vi "Pre Launch Init.vi"(11 "Keypad in":refnum<class "Keypad.lvclass">) -> (0 "error out":errorcluster, 3 "Keypad out":refnum<class "Keypad.lvclass">)   [LabVIEW 2020, in "Keypad.lvlib" / "Keypad.lvclass"]
doc: "(<B>Filename</B>: Actor Framework.lvlib:Actor.lvclass:Pre Launch Init.vi)\n\nDefines behavior that occurs after the Launch Actor method is invoked but before the actor's Actor Core method begins running.\n\nThe Pre Launch Init method is guaranteed to finish before the Launch Actor method returns to its caller and before the actor itself receives any messages. Any references that the Pre Launch Init method obtains are guaranteed to have the same lifetime as the actor itself. Any errors that the Pre Launch Init method returns will abort the launch.\n\nBy default, this method does nothing. A descendant class may override it to define behavior."
uses:
  Keypad.lvclass
  <vilib>/ni/Actors/State Actor/State Actor/State Actor.lvclass
  Type Def - Cursor Display.ctl
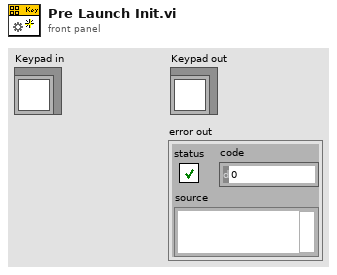
[diagram p1: front panel]
types:
  T1 = typedef "Type Def - Cursor Display.ctl" = cluster{"Up":bool, "Left":bool, "Ctr":bool, "Right":bool, "Down":bool}
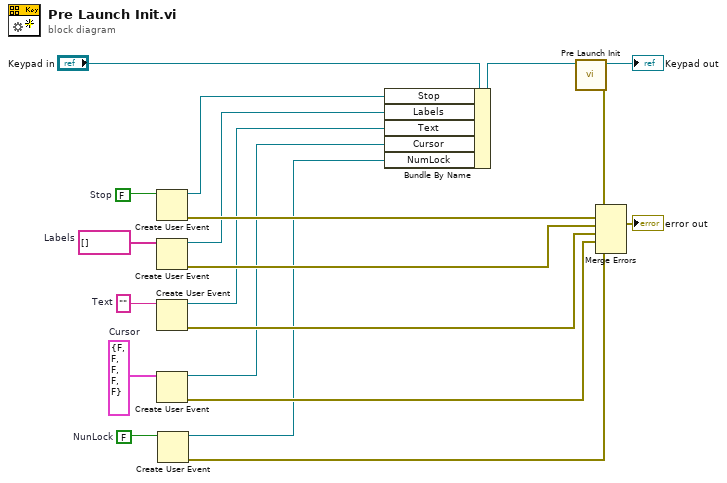
[diagram p0: block diagram]
diagram:
  w1 = T1 {"Up"=FALSE, "Left"=FALSE, "Ctr"=FALSE, "Right"=FALSE, "Down"=FALSE}  # Cursor
  w4 = FALSE  # NunLock
  w17 = ""  # Text
  w18 = FALSE  # Stop
  w19 = string[] []  # Labels
  n1 = Create User Event(user event datatype=w18) -> (user event=w10:refnum<user-event>, error out=w16:errorcluster)  [unwired: 1 in]
  n2 = Create User Event(user event datatype=w19) -> (user event=w9:refnum<user-event>, error out=w13:errorcluster)  [unwired: 1 in]
  n3 = Create User Event(user event datatype=w17) -> (user event=w8:refnum<user-event>, error out=w14:errorcluster)  [unwired: 1 in]
  n4 = Create User Event(user event datatype=w1) -> (user event=w7:refnum<user-event>, error out=w15:errorcluster)  [unwired: 1 in]
  n5 = Create User Event(user event datatype=w4) -> (user event=w3:refnum<user-event>, error out=w2:errorcluster)  [unwired: 1 in]
  n6 = Bundle By Name(cluster="Keypad in", "Stop"=w10, "Labels"=w9, "Text"=w8, "Cursor"=w7, "NumLock"=w3) -> (w5:refnum<class "Keypad.lvclass">)
  n7 = call-parent "Pre Launch Init.vi"("Actor in"=w5) -> ("error out"=w12:errorcluster, "Actor out"=→"Keypad out":refnum<class "Keypad.lvclass">)  [unwired: 9 in]
  n8 = Merge Errors(w12, w16, w13, w14, w15, w2) -> (→"error out":errorcluster)
